vi "LogEventData.vi"(8 "error in (no error)":errorcluster, 10 "eventData":refnum<class "EventData.lvclass">, 11 "EventFile in":refnum<class "EventFile.lvclass">) -> (0 "error out":errorcluster, 3 "EventFile out":refnum<class "EventFile.lvclass">)   [LabVIEW 2016, in "Event Logging.lvlib" / "EventFile.lvclass"]
uses:
  EventFile.lvclass
  EventData/EventData.lvclass
  EventFile.lvclass/EventFile.ctl
  EventData/EventData.lvclass/EventData.ctl
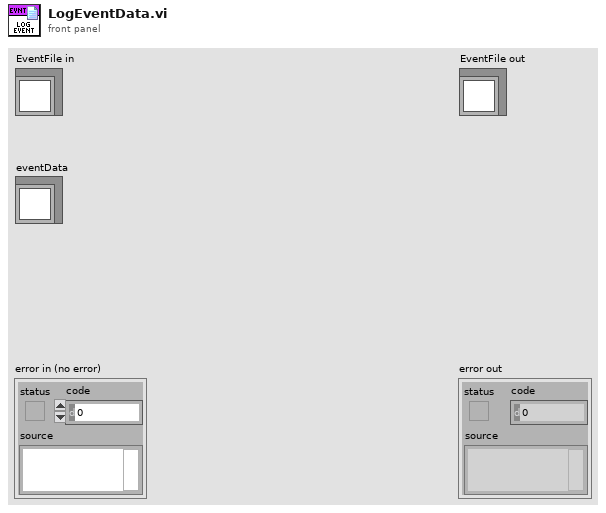
[diagram p1: front panel]
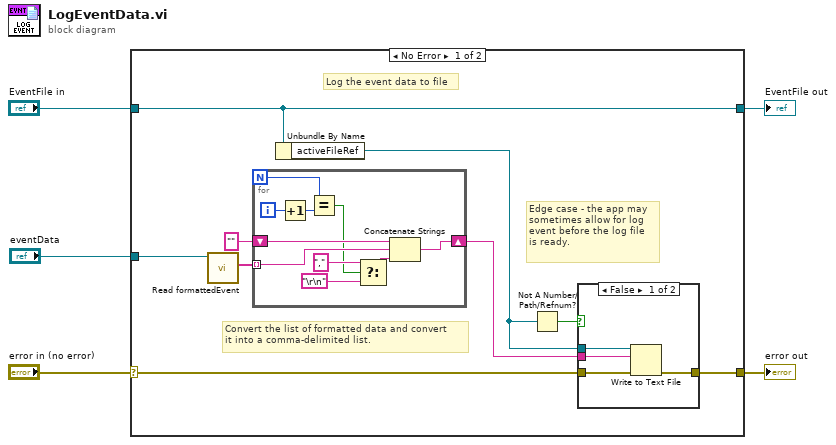
[diagram p0: block diagram]
diagram:
  n1 = case shown="No Error" "error in (no error)" {
    selector: "error in (no error)" -> [w9 w31]
    tunnel: [w8 w31] -> w4
    tunnel: [w13 w30] -> w2
    tunnel: "EventFile in" -> [w13 w30]
    tunnel: "eventData" -> [w14 _]
    frame No Error {
      # "Edge case - the app may\nsometimes allow for log\nevent before the log file\nis ready."
      # "Convert the list of formatted data and convert\nit into a comma-delimited list."
      # "Log the event data to file"
      n2 = call "Read formattedEvent.vi"("EventData in"=w14) -> ("formattedEvent"=w12:string[])  [unwired: 8 in, 2 out]
      n3 = for {
        N -> [w24]
        tunnel: w12 -> [w28] mode=indexing
        shift-right: [w27] -> w10
        shift-left: "" -> [w29]
        i -> [w26]
        n4 = Increment(x=w26) -> (x+1=w25:i32)
        n5 = Equal?(x=w24, y=w25) -> (x = y?=w21:bool)
        n6 = Select(t=",", s=w21, f="\r\n") -> (s? t:f=w20:string)
        n7 = Concatenate Strings(w29, w28, w20) -> (w27:string)
      }
      n8 = Unbundle By Name(w13) -> ("activeFileRef"=w7:refnum<file>)
      n9 = Not A Number/Path/Refnum?(number/path/refnum=w7) -> (NaN/Path/Refnum?=w6:bool)
      n10 = case shown="False" w6 {
        tunnel: w10 -> [w18 _]
        tunnel: w9 -> [w17 w19]
        tunnel: [w16 w19] -> w8
        tunnel: w7 -> [w15 _]
        frame False {
          n11 = Write to Text File(file (use dialog)=w15, text=w18, error in=w17) -> (error out=w16:errorcluster)  [unwired: 1 in, 2 out]
        }
        frame True {
        }
      }
    }
    frame Error {
    }
  }
  "error out" <- w4
  "EventFile out" <- w2
